vi "POP_FG.Popup.vi"(0 "Popup Parameters":T1, 1 "Popup Operation":T4, 2 "Name":string, 3 "TontName":string="Tahoma", 5 "Encoded Location":string, 9 "Font Size":u32, 11 "Error In":errorcluster caption="错误输入（无错误）", 12 "Popup Ref":refnum<vi>, 14 "Popup Accepted?":bool) -> (4 "Event":refnum<user-event>, 6 "Popup Parameters out":T1={"Prop Type"=enum."Unkown", "Initial Value"=variant, "Caption Strings"=[], "Ring Strings"=[], "Cell Rect"={"left"=0, "top"=0, "right"=0, "bottom"=0}, "Mouse Coords"={"x"=0, "y"=0}, "Call Data"=variant, "Ring Values"=[], "Browse Options"={"Prompt"="", "Match Pattern"="", "Mode"=enum."existing file", "Start Path"=path "", "Pattern Label"="", "Button Text"=""}, "Combo Box"={"Allow Undefined Strings"=FALSE}}, 10 "Found":bool, 15 "Error Out":errorcluster caption="错误输入（无错误）")   [LabVIEW 2016]
uses:
  Ctrls/POP_Popup Operation.ctl
  Ctrls/POP_Popup Results.ctl
  Ctrls/POP_Popup Call Parameters.ctl
  Ctrls/POP_Data Type.ctl
  <vilib>/Utility/miscctls.llb/LVBrowseOptionsTypeDef.ctl
  Ctrls/POP_Core Data.ctl
  Ctrls/POP_Monitor Register Data.ctl
  Ctrls/POP_Event Enum.ctl
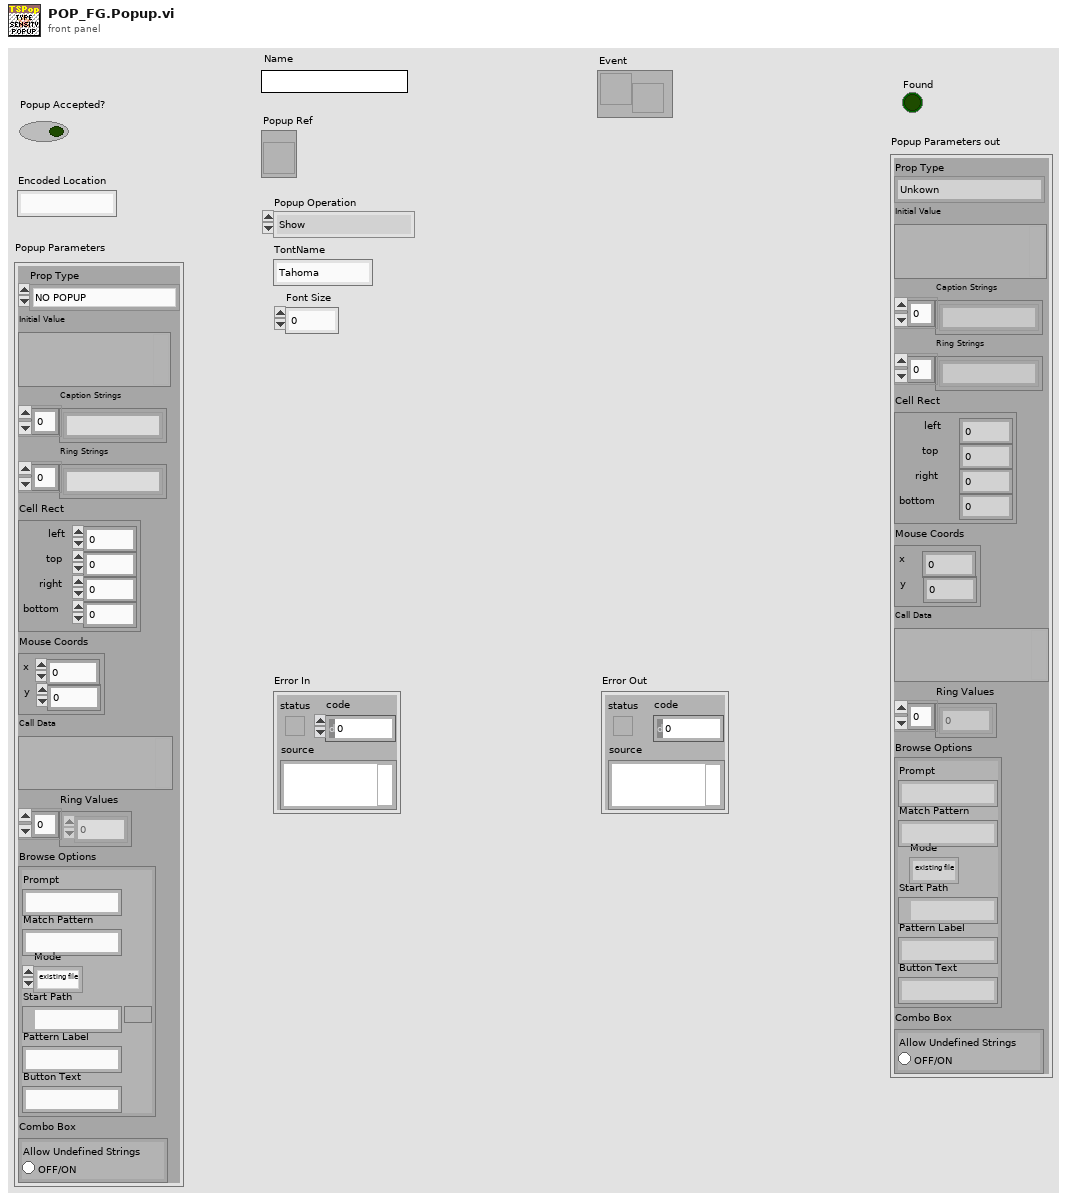
[diagram p1: front panel]
types:
  T1 = typedef "POP_Popup Call Parameters.ctl" = cluster{"Prop Type":T2, "Initial Value":variant, "Caption Strings":string[], "Ring Strings":string[], "Cell Rect":cluster{"left":i16, "top":i16, "right":i16, "bottom":i16}, "Mouse Coords":cluster{"x":i16, "y":i16}, "Call Data":variant, "Ring Values":ext[], "Browse Options":T3, "Combo Box":cluster{"Allow Undefined Strings":bool}}
  T2 = typedef "POP_Data Type.ctl" = enum16{"NO POPUP", "Unkown", "String", "Integer", "Float", "Color", "Boolean", "Ring", "Captioned String", "Captioned Integer", "Button Color", "2 Int Cluster", "4 Int Cluster", "6-Dbl Cluster", "Path", "Combox", "Time", "ShotCut String"}
  T3 = typedef "LVBrowseOptionsTypeDef.ctl" = cluster{"Prompt":string, "Match Pattern":string, "Mode":enum32{"existing file", "new file", "new or existing file", "existing dir", "new dir", "new or existing dir", "existing file (use LLBs)", "new file (use LLBs)", "new or existing file (use LLBs)", "new or existing file or directory (use LLBs)", "existing dir (use LLBs)", "new dir (use LLBs)", "new or existing dir (use LLBs)", "existing file or dir", "new file or dir", "new or existing file or dir", "existing file or dir (use LLBs)", "new file or dir (use LLBs)"}, "Start Path":path, "Pattern Label":string, "Button Text":string}
  T4 = typedef "POP_Popup Operation.ctl" = enum16{"Show", "Initialize", "Close", "Popup Done", "Register a Location's Type", "Retrieve Location's Type"}
  T5 = typedef "POP_Core Data.ctl" = cluster{"Quit Evt":refnum<user-event>, "Reg Evt":refnum<user-event>, "Done Evt":refnum<user-event>, "Popup Ref":refnum<vi>, "Event Data":T6, "Offsets":cluster{"Left":i32, "Top":i32}[], "Reg Type":variant, "Popup Parameters":T1, "LV Version":string}
  T6 = typedef "POP_Monitor Register Data.ctl" = cluster{"Control":refnum<vi>, "Events":T7[]}
  T7 = typedef "POP_Event Enum.ctl" = enum16{"Nothing", "Enter Key Accept", "Escape Key Cancel", "Mouse Outside Accept", "Mouse Outside Cancel", "Mouse Move Accept", "Mouse Move Cancel", "Mouse Leave Cancel", "Value Change Accept", "Lose Focus Cancel", "Cancel Button", "Accept Button", "Shift Ctrl Key Down"}
  T8 = typedef "POP_Popup Results.ctl" = cluster{"Valid?":bool, "Value Changed?":bool, "Popup Value":variant, "Call Data":variant}
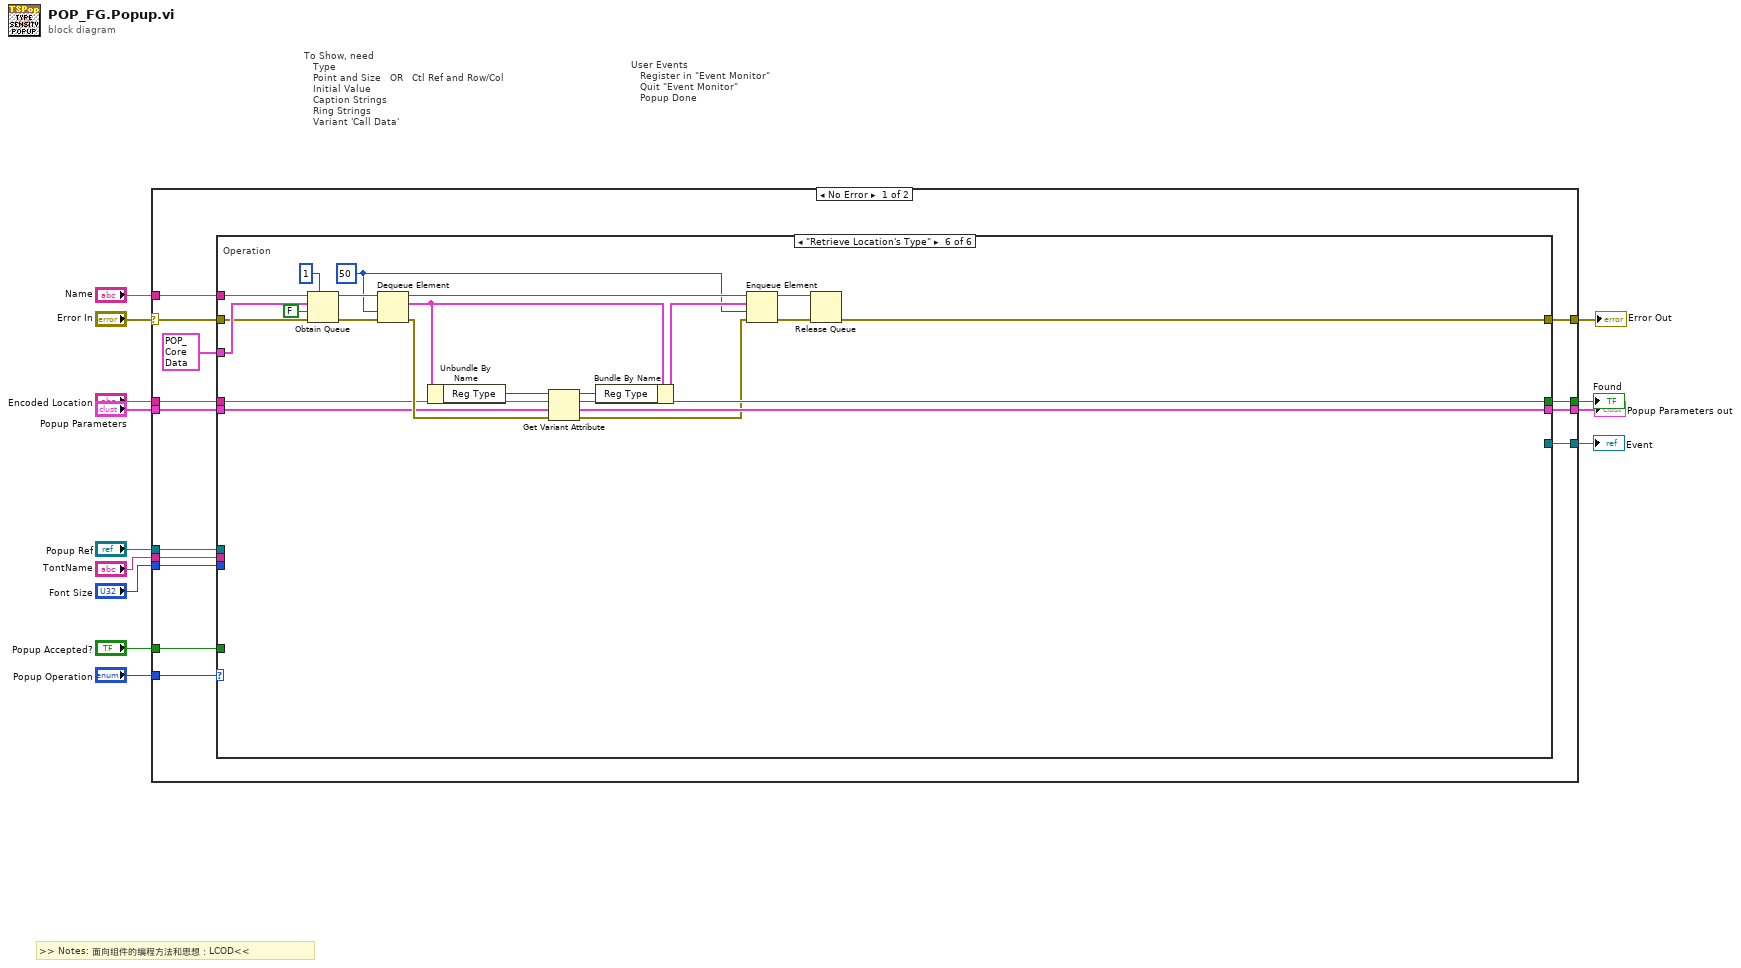
[diagram p0: block diagram]
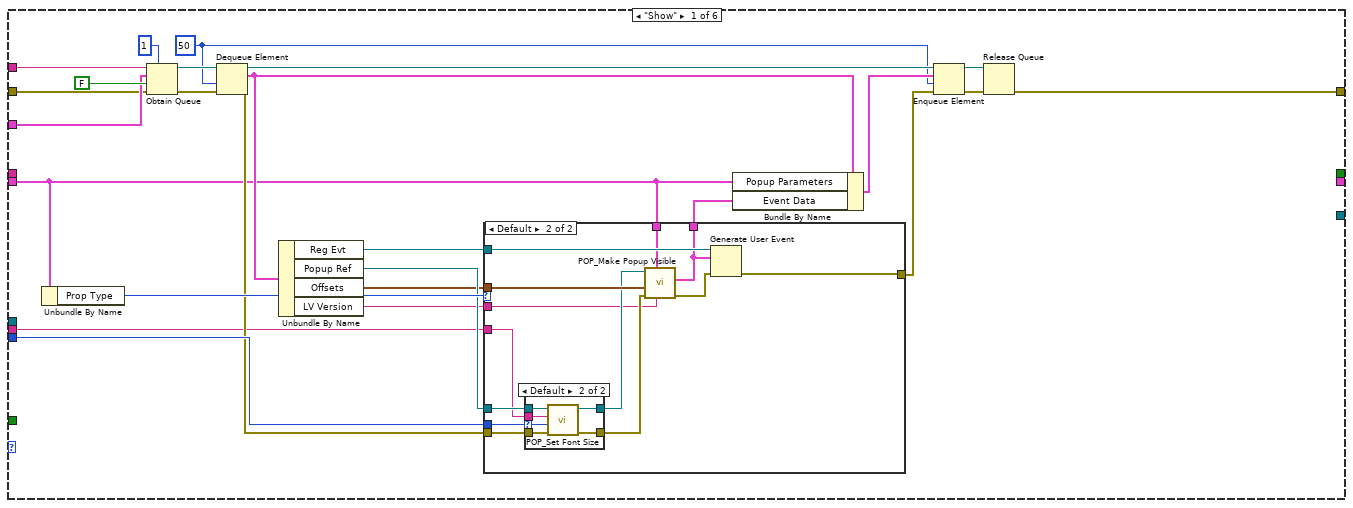
[diagram p2: hidden frame]
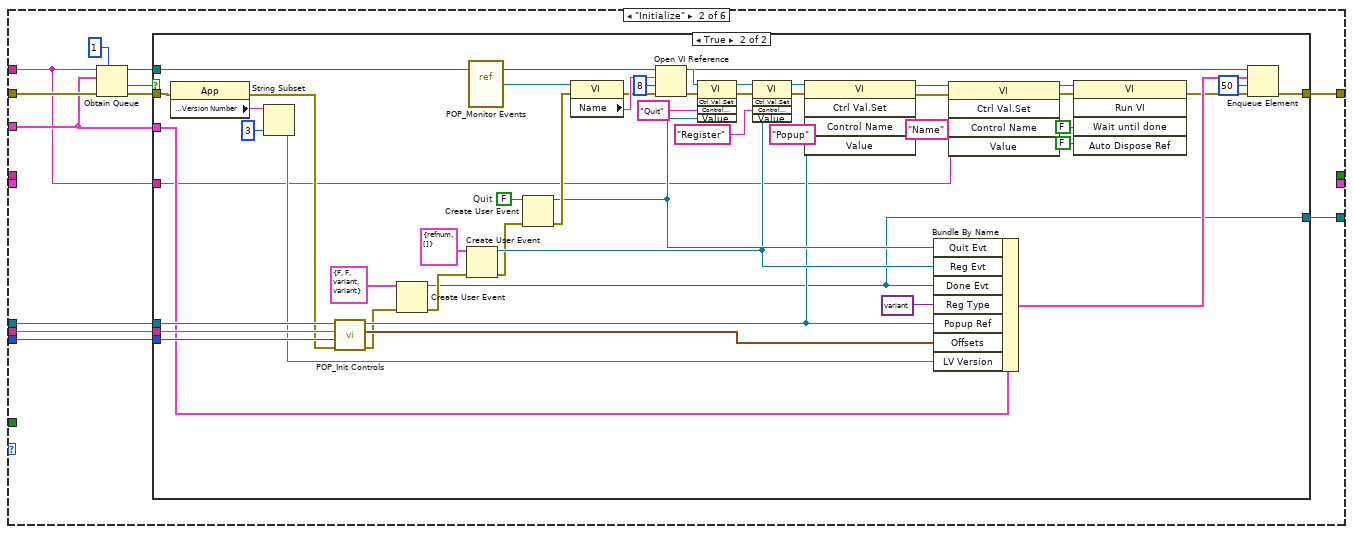
[diagram p5: hidden frame]
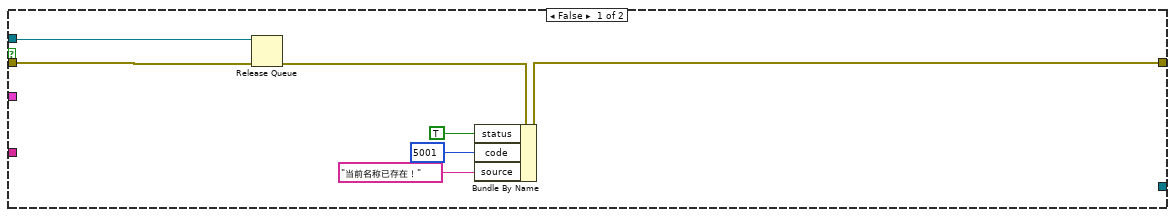
[diagram p6: hidden frame]
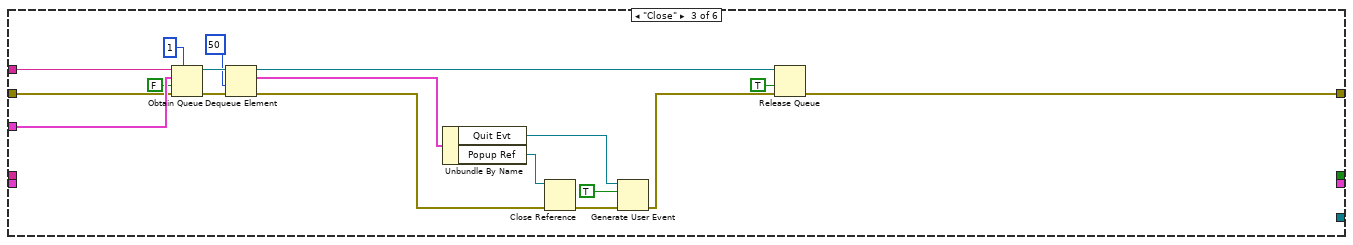
[diagram p7: hidden frame]
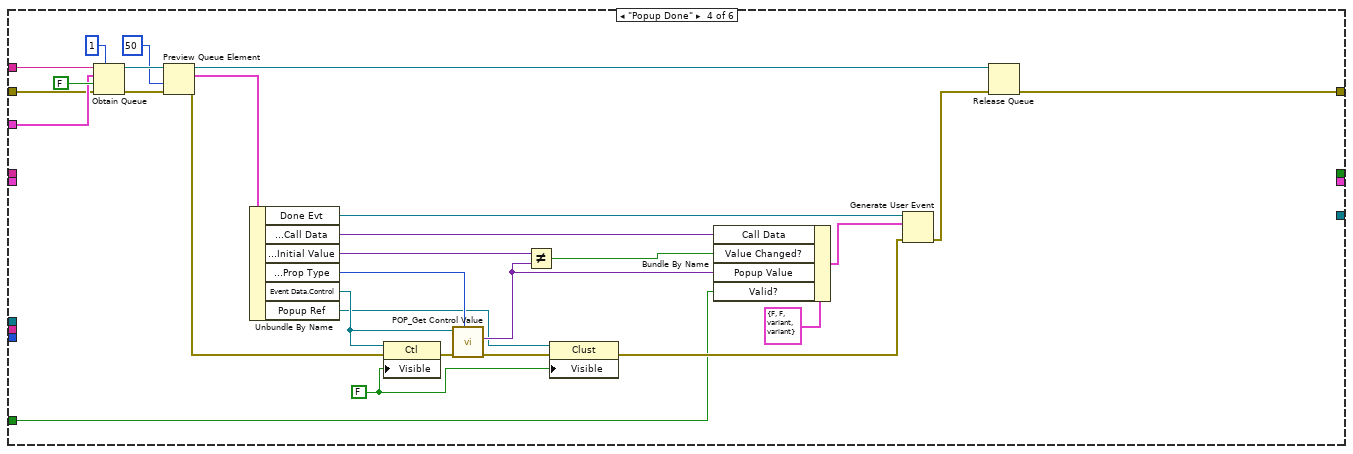
[diagram p8: hidden frame]
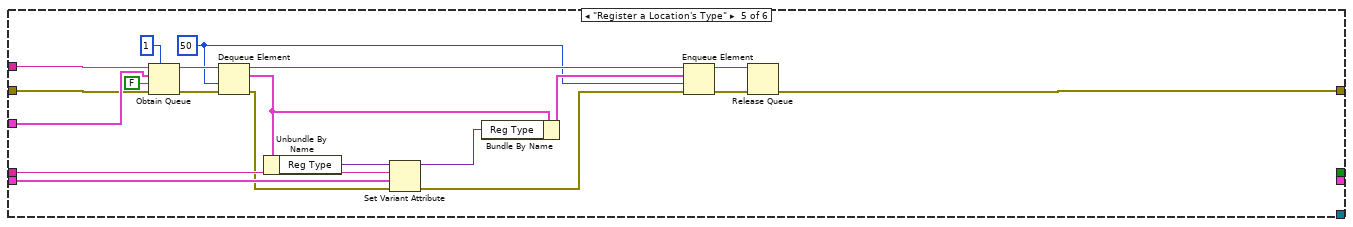
[diagram p9: hidden frame]
diagram:
  # ">> Notes: 面向组件的编程方法和思想：LCOD<<"
  # "User Events\n   Register in \"Event Monitor\"\n   Quit \"Event Monitor\"\n   Popup Done"
  # "To Show, need\n   Type\n   Point and Size   OR   Ctl Ref and Row/Col\n   Initial Value\n   Caption Strings\n   Ring Strings\n   Variant 'Call Data'"
  n1 = case shown="No Error" "Error In" {
    selector: "Error In" -> [w18 w230]
    tunnel: [w17 w230] -> w2
    tunnel: "Popup Operation" -> [w27 _]
    tunnel: [w26 _] -> w12
    tunnel: "Popup Parameters" -> [w23 _]
    tunnel: "Popup Ref" -> [w25 _]
    tunnel: "Popup Accepted?" -> [w24 _]
    tunnel: "Encoded Location" -> [w22 _]
    tunnel: [w21 _] -> w7
    tunnel: [w20 _] -> w6
    tunnel: "Font Size" -> [w19 _]
    tunnel: "TontName" -> [w16 _]
    tunnel: "Name" -> [w15 _]
    frame No Error {
      n2 = case "Operation" shown="\"Retrieve Location's Type\"" w27 {
        tunnel: [_ w86 _ _ _ _] -> w26
        tunnel: w25 -> [_ w84 _ _ _ _]
        tunnel: w24 -> [_ _ _ w160 _ _]
        tunnel: w23 -> [w36 _ _ _ w206 w214]
        tunnel: w22 -> [_ _ _ _ w207 w215]
        tunnel: [_ _ _ _ _ w213] -> w21
        tunnel: [_ _ _ _ _ w212] -> w20
        tunnel: w19 -> [w52 w85 _ _ _ _]
        tunnel: w18 -> [w42 w80 w153 w165 w198 w208]
        tunnel: [w40 w82 w144 w163 w188 w209] -> w17
        tunnel: w16 -> [w28 w83 _ _ _ _]
        tunnel: w15 -> [w46 w75 w156 w176 w201 w218]
        tunnel: T5 {"Quit Evt"=refnum, "Reg Evt"=refnum, "Done Evt"=refnum, "Popup Ref"=refnum, "Event Data"={"Control"=refnum, "Events"=[]}, "Offsets"=[], "Reg Type"=variant, "Popup Parameters"={"Prop Type"=enum."NO POPUP", "Initial Value"=variant, "Caption Strings"=[], "Ring Strings"=[], "Cell Rect"={"left"=0, "top"=0, "right"=0, "bottom"=0}, "Mouse Coords"={"x"=0, "y"=0}, "Call Data"=variant, "Ring Values"=[], "Browse Options"={"Prompt"="", "Match Pattern"="", "Mode"=enum."existing file", "Start Path"=path "", "Pattern Label"="", "Button Text"=""}, "Combo Box"={"Allow Undefined Strings"=FALSE}}, "LV Version"=""} ("Data") -> [w45 w76 w155 w175 w200 w219]
        frame "Show" {
          w30 = 50 ("超时毫秒(-1)")
          n3 = Unbundle By Name(w36) -> ("Prop Type"=w51:T2)
          n4 = Obtain Queue(max queue size (-1, unlimited)=1 ("队列最大值（-1，无限）"), name (unnamed)=w46, element data type=w45, create if not found? (T)=FALSE ("如未找到是否创建？(T)"), error in (no error)=w42) -> (queue out=w47:refnum<queue>, error out=w48:errorcluster)  [unwired: 1 out]
          n5 = Dequeue Element(queue=w47, timeout in ms (-1)=w30, error in (no error)=w48) -> (queue out=w35:refnum<queue>, element=w37:T5, error out=w41:errorcluster)  [unwired: 1 out]
          n6 = Unbundle By Name(w37) -> ("Reg Evt"=w44:refnum<user-event>, "Popup Ref"=w43:refnum<vi>, "Offsets"=w38:cluster{"Left":i32, "Top":i32}[], "LV Version"=w39:string)
          n7 = case shown="Default" w51 {
            tunnel: w44 -> [_ w66]
            tunnel: w38 -> [_ w65]
            tunnel: w36 -> [_ w64]
            tunnel: w52 -> [_ w63]
            tunnel: w43 -> [_ w62]
            tunnel: w41 -> [w53 w59]
            tunnel: [w53 w57] -> w33
            tunnel: w39 -> [_ w56]
            tunnel: [_ w55] -> w29
            tunnel: w28 -> [_ w54]
            frame "NO POPUP" {
            }
            frame Default {
              n8 = case shown="Default" w63 {
                selector: w63 -> [_ w74]
                tunnel: w62 -> [w68 w73]
                tunnel: [w68 w72] -> w61
                tunnel: w59 -> [w67 w71]
                tunnel: [w67 w70] -> w58
                tunnel: w54 -> [_ w69]
                frame 0 {
                }
                frame Default {
                  n9 = call "POP_Set Font Size.vi"("error in (no error)"=w71, "Font Size"=w74, "TontName"=w69, "Popup Cluster Ref"=w73) -> ("error out"=w70:errorcluster, "dup ref out"=w72:refnum<vi>)  [unwired: 6 in]
                }
              }
              n10 = call "POP_Make Popup Visible.vi"("LV Version"=w56, "Popup Parameters"=w64, "error in (no error)"=w58, "Ctl Offsets"=w65, "Popup Cluster Ref"=w61) -> ("error out"=w60:errorcluster, "event data"=w55:T6)  [unwired: 5 in]
              n11 = Generate User Event(user event=w66, event data cluster=w55, error in=w60) -> (error out=w57:errorcluster)  [unwired: 1 in, 1 out]
            }
          }
          n12 = Bundle By Name(cluster=w37, "Popup Parameters"=w36, "Event Data"=w29) -> (w31:T5)
          n13 = Enqueue Element(queue=w35, element=w31, timeout in ms (-1)=w30, error in (no error)=w33) -> (queue out=w34:refnum<queue>, error out=w32:errorcluster)  [unwired: 1 out]
          n14 = Release Queue(queue=w34, error in (no error)=w32) -> (error out=w40:errorcluster)  [unwired: 1 in, 2 out]
        }
        frame "Initialize" {
          n15 = Obtain Queue(max queue size (-1, unlimited)=1 ("队列最大值（-1，无限）"), name (unnamed)=w75, element data type=w76, error in (no error)=w80) -> (queue out=w77:refnum<queue>, created new?=w78:bool, error out=w79:errorcluster)  [unwired: 1 in]
          n16 = case shown="True" w78 {
            tunnel: [_ w100] -> w86
            tunnel: w85 -> [_ w127]
            tunnel: w84 -> [_ w126]
            tunnel: w83 -> [_ w125]
            tunnel: [w88 w110] -> w82
            tunnel: w79 -> [w89 w103]
            tunnel: w77 -> [w87 w117]
            tunnel: w76 -> [_ w116]
            tunnel: w75 -> [_ w95]
            frame False {
              n17 = Release Queue(queue=w87, error in (no error)=w89) -> (error out=w90:errorcluster)  [unwired: 1 in, 2 out]
              n18 = Bundle By Name(cluster=w90, "status"=TRUE, "code"=5001, "source"="当前名称已存在！") -> (w88:errorcluster)
            }
            frame True {
              w140 = FALSE  # Quit
              n19 = property class="App"(error in=w103) -> (error out=w104:errorcluster, "Application:Version Number"=w129:string)  [unwired: 1 in, 1 out]
              n20 = String Subset(string=w129, length (rest)=3 ("length")) -> (substring=w102:string)  [unwired: 1 in]
              n21 = call "POP_Init Controls.vi"("Error In"=w104, "Font Size"=w127, "TontName"=w125, "Popup Cluster Ref"=w126) -> ("Error Out"=w101:errorcluster, "Offsets"=w109:cluster{"Left":i32, "Top":i32}[], "Popup Cluster Ref Out"=w113:refnum<vi>)  [unwired: 5 in]
              n22 = Create User Event(user event datatype=T8 {"Valid?"=FALSE, "Value Changed?"=FALSE, "Popup Value"=variant, "Call Data"=variant} ("Popup Results (type only)"), error in=w101) -> (user event=w100:refnum<user-event>, error out=w105:errorcluster)
              n23 = Create User Event(user event datatype=T6 {"Control"=refnum, "Events"=[]} ("Reg. Data (type only)"), error in=w105) -> (user event=w114:refnum<user-event>, error out=w106:errorcluster)
              n24 = vi-ref "POP_Monitor Events.vi"() -> (w121:refnum<vi>)
              n25 = Create User Event(user event datatype=w140, error in=w106) -> (user event=w115:refnum<user-event>, error out=w118:errorcluster)
              n26 = property class="VI"(reference=w121, error in=w118) -> (error out=w119:errorcluster, "Name"=w120:string)  [unwired: 1 out]
              n27 = Open VI Reference(vi path=w120, options=8 ("选项"), error in (no error)=w119) -> (vi reference=w124:refnum<vi>, error out=w122:errorcluster)  [unwired: 3 in]
              n28 = invoke on="Set Control (Variant)" class="VI" method="Ctrl Val.Set"(reference=w124, error in=w122, "Control Name"="Quit", "Value"=w115) -> (reference out=w134:refnum<vi>, error out=w135:errorcluster)  [unwired: 1 in, 3 out]
              n29 = invoke on="Set Control (Variant)" class="VI" method="Ctrl Val.Set"(reference=w134, error in=w135, "Control Name"="Register", "Value"=w114) -> (reference out=w132:refnum<vi>, error out=w133:errorcluster)  [unwired: 1 in, 3 out]
              n30 = invoke on="Set Control (Variant)" class="VI" method="Ctrl Val.Set"(reference=w132, error in=w133, "Control Name"="Popup", "Value"=w113) -> (reference out=w99:refnum<vi>, error out=w96:errorcluster)  [unwired: 1 in, 3 out]
              n31 = Bundle By Name(cluster=w116, "Quit Evt"=w115, "Reg Evt"=w114, "Done Evt"=w100, "Reg Type"=variant ("Variant"), "Popup Ref"=w113, "Offsets"=w109, "LV Version"=w102) -> (w112:T5)
              n32 = invoke on="Set Control (Variant)" class="VI" method="Ctrl Val.Set"(reference=w99, error in=w96, "Control Name"="Name", "Value"=w95) -> (reference out=w98:refnum<vi>, error out=w97:errorcluster)  [unwired: 1 in, 3 out]
              n33 = invoke class="VI" method="Run VI"(reference=w98, error in=w97, "Wait until done"=FALSE, "Auto Dispose Ref"=FALSE ("Wait until done")) -> (error out=w107:errorcluster)  [unwired: 1 in, 4 out]
              n34 = Enqueue Element(queue=w117, element=w112, timeout in ms (-1)=50 ("超时毫秒(-1)"), error in (no error)=w107) -> (error out=w110:errorcluster)  [unwired: 2 out]
            }
          }
        }
        frame "Close" {
          n35 = Obtain Queue(max queue size (-1, unlimited)=1 ("队列最大值（-1，无限）"), name (unnamed)=w156, element data type=w155, create if not found? (T)=FALSE ("如未找到是否创建？(T)"), error in (no error)=w153) -> (queue out=w151:refnum<queue>, error out=w152:errorcluster)  [unwired: 1 out]
          n36 = Dequeue Element(queue=w151, timeout in ms (-1)=50 ("超时毫秒(-1)"), error in (no error)=w152) -> (queue out=w143:refnum<queue>, element=w149:T5, error out=w146:errorcluster)  [unwired: 1 out]
          n37 = Unbundle By Name(w149) -> ("Quit Evt"=w148:refnum<user-event>, "Popup Ref"=w147:refnum<vi>)
          n38 = Close Reference(reference=w147, error in (no error)=w146) -> (error out=w158:errorcluster)
          n39 = Generate User Event(user event=w148, event data cluster=TRUE ("event data"), error in=w158) -> (error out=w145:errorcluster)  [unwired: 1 in, 1 out]
          n40 = Release Queue(queue=w143, force destroy? (F)=TRUE ("强制销毁？(F)"), error in (no error)=w145) -> (error out=w144:errorcluster)  [unwired: 2 out]
        }
        frame "Popup Done" {
          w185 = FALSE ("Visible")
          n41 = Obtain Queue(max queue size (-1, unlimited)=1 ("队列最大值（-1，无限）"), name (unnamed)=w176, element data type=w175, create if not found? (T)=FALSE ("如未找到是否创建？(T)"), error in (no error)=w165) -> (queue out=w177:refnum<queue>, error out=w178:errorcluster)  [unwired: 1 out]
          n42 = Preview Queue Element(queue=w177, timeout in ms (-1)=50 ("超时毫秒(-1)"), error in (no error)=w178) -> (queue out=w168:refnum<queue>, element=w174:T5, error out=w164:errorcluster)  [unwired: 1 out]
          n43 = Unbundle By Name(w174) -> ("Done Evt"=w162:refnum<user-event>, "Popup Parameters.Call Data"=w161:variant, "Popup Parameters.Initial Value"=w173:variant, "Popup Parameters.Prop Type"=w172:T2, "Event Data.Control"=w171:refnum<vi>, "Popup Ref"=w170:refnum<vi>)
          n44 = property on="Property Node" class="Ctl"(reference=w171, error in=w164, "Visible"=w185) -> (error out=w183:errorcluster)  [unwired: 1 out]
          n45 = call "POP_Get Control Value.vi"("Prop Type"=w172, "error in (no error)"=w183, "Control"=w171) -> ("error out"=w182:errorcluster, "Value"=w184:variant)  [unwired: 6 in, 1 out]
          n46 = Not Equal?(x=w173, y=w184) -> (x != y?=w186:bool)
          n47 = property class="Clust"(reference=w170, error in=w182, "Visible"=w185) -> (error out=w181:errorcluster)  [unwired: 1 out]
          n48 = Bundle By Name(cluster=T8 {"Valid?"=FALSE, "Value Changed?"=FALSE, "Popup Value"=variant, "Call Data"=variant} ("Popup Results (type only)"), "Call Data"=w161, "Value Changed?"=w186, "Popup Value"=w184, "Valid?"=w160) -> (w187:T8)
          n49 = Generate User Event(user event=w162, event data cluster=w187, error in=w181) -> (error out=w166:errorcluster)  [unwired: 1 in, 1 out]
          n50 = Release Queue(queue=w168, error in (no error)=w166) -> (error out=w163:errorcluster)  [unwired: 1 in, 2 out]
        }
        frame "Register a Location's Type" {
          w192 = 50 ("超时毫秒(-1)")
          n51 = Obtain Queue(max queue size (-1, unlimited)=1 ("队列最大值（-1，无限）"), name (unnamed)=w201, element data type=w200, create if not found? (T)=FALSE ("如未找到是否创建？(T)"), error in (no error)=w198) -> (queue out=w202:refnum<queue>, error out=w203:errorcluster)  [unwired: 1 out]
          n52 = Dequeue Element(queue=w202, timeout in ms (-1)=w192, error in (no error)=w203) -> (queue out=w194:refnum<queue>, element=w196:T5, error out=w197:errorcluster)  [unwired: 1 out]
          n53 = Unbundle By Name(w196) -> ("Reg Type"=w199:variant)
          n54 = Set Variant Attribute(Variant=w199, name=w207, value=w206, error in=w197) -> (Variant out=w195:variant, error out=w191:errorcluster)  [unwired: 1 out]
          n55 = Bundle By Name(cluster=w196, "Reg Type"=w195) -> (w193:T5)
          n56 = Enqueue Element(queue=w194, element=w193, timeout in ms (-1)=w192, error in (no error)=w191) -> (queue out=w190:refnum<queue>, error out=w189:errorcluster)  [unwired: 1 out]
          n57 = Release Queue(queue=w190, error in (no error)=w189) -> (error out=w188:errorcluster)  [unwired: 1 in, 2 out]
        }
        frame "Retrieve Location's Type" {
          w222 = 50 ("超时毫秒(-1)")
          n58 = Obtain Queue(max queue size (-1, unlimited)=1 ("队列最大值（-1，无限）"), name (unnamed)=w218, element data type=w219, create if not found? (T)=FALSE ("如未找到是否创建？(T)"), error in (no error)=w208) -> (queue out=w226:refnum<queue>, error out=w227:errorcluster)  [unwired: 1 out]
          n59 = Dequeue Element(queue=w226, timeout in ms (-1)=w222, error in (no error)=w227) -> (queue out=w224:refnum<queue>, element=w225:T5, error out=w216:errorcluster)  [unwired: 1 out]
          n60 = Unbundle By Name(w225) -> ("Reg Type"=w217:variant)
          n61 = Get Variant Attribute(Variant=w217, name=w215, default value (empty Variant)=w214, error in=w216) -> (duplicate Variant=w211:variant, found=w213:bool, value=w212:T1, error out=w210:errorcluster)
          n62 = Bundle By Name(cluster=w225, "Reg Type"=w211) -> (w223:T5)
          n63 = Enqueue Element(queue=w224, element=w223, timeout in ms (-1)=w222, error in (no error)=w210) -> (queue out=w221:refnum<queue>, error out=w220:errorcluster)  [unwired: 1 out]
          n64 = Release Queue(queue=w221, error in (no error)=w220) -> (error out=w209:errorcluster)  [unwired: 1 in, 2 out]
        }
      }
    }
    frame Error {
    }
  }
  "Event" <- w12
  "Found" <- w7
  "Popup Parameters out" <- w6
  "Error Out" <- w2
